vi "Advance past String.vi"(7 "JSON":string, 9 "Offset":i32, 11 "State in":T1=enum."String") -> (1 "Offset past match":i32, 3 "State":T1, 6 "Value start out":i32)   [LabVIEW 2024, in "JSONtext.lvlib"]
uses:
  JSONtext.lvlib
  Parsing State.ctl
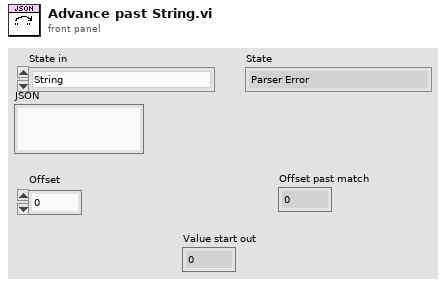
[diagram p1: front panel]
types:
  T1 = typedef "JSONtext.lvlib/Parsing State.ctl" = enum16{"Parser Error", "Object", "Array", "String", "Number/Other", "Leading Whitespace", "Object end", "Array end", "Value end"}
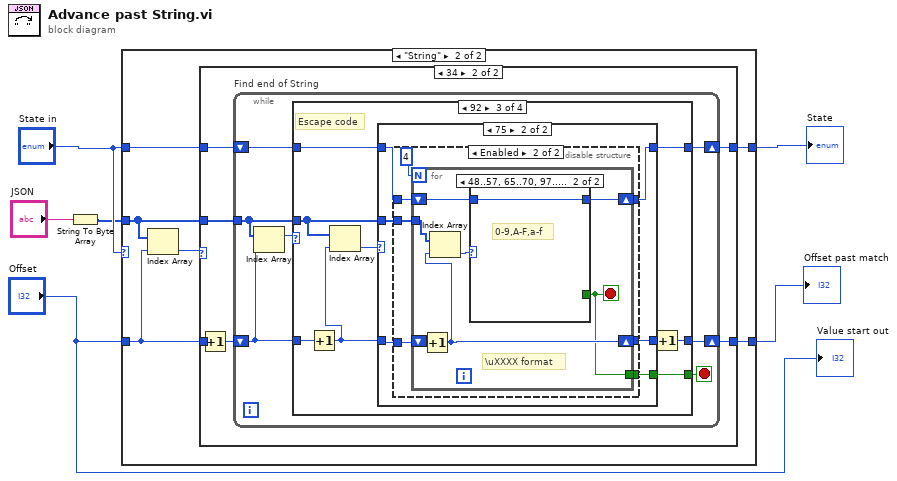
[diagram p0: block diagram]
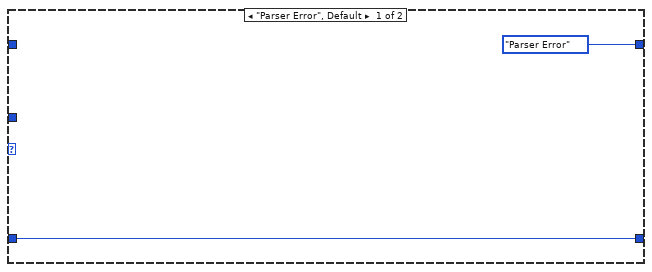
[diagram p2: hidden frame]
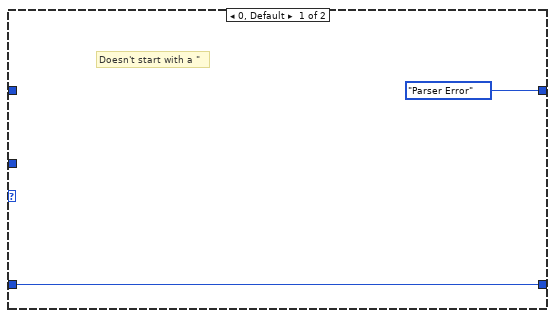
[diagram p3: hidden frame]
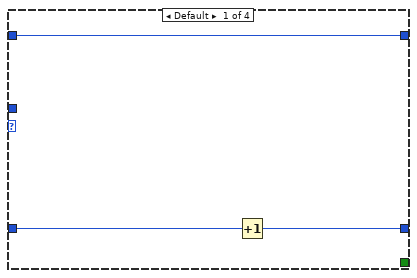
[diagram p4: hidden frame]
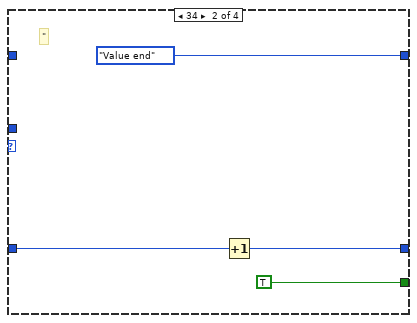
[diagram p5: hidden frame]
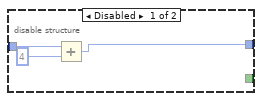
[diagram p7: hidden frame]
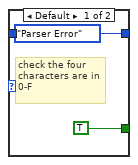
[diagram p8: hidden frame]
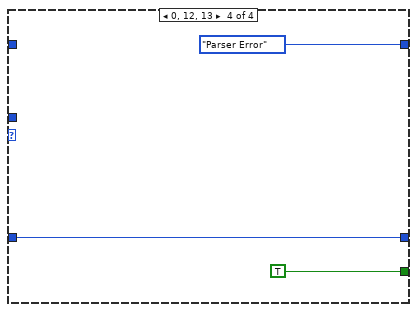
[diagram p9: hidden frame]
diagram:
  n1 = String To Byte Array(string="JSON") -> (unsigned byte array=w1:u8[])
  n2 = case shown="\"String\"" "State in" {
    tunnel: [Parsing_State."Parser Error" ("State in") w14] -> w6
    tunnel: [w8 w13] -> w5
    tunnel: w1 -> [_ w11]
    tunnel: "State in" -> [_ w12]
    tunnel: "Offset" -> [w8 w10]
    frame "Parser Error", Default {
    }
    frame "String" {
      n3 = Index Array(array=w11, index=w10) -> (element=w9:u8)
      n4 = case shown="34" w9 {
        tunnel: [Parsing_State."Parser Error" ("State in") w22] -> w14
        tunnel: [w15 w21] -> w13
        tunnel: w12 -> [_ w20]
        tunnel: w11 -> [_ w18]
        tunnel: w10 -> [w15 w17]
        frame 0, Default {
          # "Doesn't start with a \""
        }
        frame 34 {
          n5 = Increment(x=w17) -> (x+1=w19:i32)
          n6 = while "Find end of String" {
            tunnel: w18 -> [w28]
            shift-right: [w23] -> w21
            shift-left: w19 -> [w24]
            shift-right: [w26] -> w22
            shift-left: w20 -> [w27]
            stop <- w25 stop-if-true
            n7 = Index Array(array=w28, index=w24) -> (element=w29:u8)
            n8 = case shown="92" w29 {
              tunnel: w28 -> [_ _ w38 _]
              tunnel: w27 -> [w32 _ w39 _]
              tunnel: [w32 Parsing_State."Value end" w40 Parsing_State."Parser Error"] -> w26
              tunnel: [_ TRUE w37 TRUE] -> w25
              tunnel: w24 -> [w31 w34 w45 w76]
              tunnel: [w30 w33 w41 w76] -> w23
              frame Default {
                n9 = Increment(x=w31) -> (x+1=w30:i32)
              }
              frame 34 {
                # "\""
                n10 = Increment(x=w34) -> (x+1=w33:i32)
              }
              frame 92 {
                # "Escape code"
                n11 = Increment(x=w45) -> (x+1=w43:i32)
                n12 = Index Array(array=w38, index=w43) -> (element=w44:u8)
                n13 = case shown="75" w44 {
                  tunnel: w43 -> [w47 w53]
                  tunnel: [w47 w52] -> w42
                  tunnel: [w46 w49] -> w40
                  tunnel: w39 -> [w46 w50]
                  tunnel: w38 -> [_ w51]
                  tunnel: [_ w48] -> w37
                  frame Default {
                    # "escaped character"
                  }
                  frame 117 {
                    n14 = disable-structure shown="Enabled" {
                      disable-tunnel: w53 -> [w56 w63]
                      disable-tunnel: [w54 w59] -> w52
                      disable-tunnel: w51 -> [_ w61]
                      disable-tunnel: w50 -> [_ w60]
                      disable-tunnel: [_ w58] -> w49
                      disable-tunnel: [_ w57] -> w48
                      frame Disabled {
                        n15 = Add(x=w56, y=4) -> (x+y=w54:i32)
                      }
                      frame Enabled {
                        n16 = for {
                          N: 4 -> [_]
                          tunnel: w61 -> [w68]
                          shift-right: [w66] -> w58
                          shift-left: w60 -> [w67]
                          shift-right: [w65] -> w59
                          shift-left: w63 -> [w70]
                          tunnel: [w64] -> w57
                          stop <- w64 stop-if-true
                          # "\\uXXXX format"
                          n17 = Increment(x=w70) -> (x+1=w65:i32)
                          n18 = Index Array(array=w68, index=w65) -> (element=w69:u8)
                          n19 = case shown="48..57, 65..70, 97..102" w69 {
                            tunnel: w67 -> [_ w73]
                            tunnel: [Parsing_State."Parser Error" ("State in") w73] -> w66
                            tunnel: [TRUE _] -> w64
                            frame Default {
                              # "check the four\ncharacters are in\n0-F"
                            }
                            frame 48..57, 65..70, 97..102 {
                              # "0-9,A-F,a-f"
                            }
                          }
                        }
                      }
                    }
                  }
                }
                n20 = Increment(x=w42) -> (x+1=w41:i32)
              }
              frame 0, 12, 13 {
              }
            }
          }
        }
      }
    }
  }
  "State" <- w6
  "Offset past match" <- w5
  "Value start out" <- "Offset"
